vi "AttackerNormal.vi"(4 "AI Parameters":T1={"GotoKick"={"Dist do cone a frente"=150.0, "attacker farback"=1500.0, "Perto"=300.0, "min dist to kick"=150.0, "kick eps"=0.05, "Time to transition"=0.0}, "Attacker"={"CC chute"=0.09, "CC passe"=0.045, "Kick Force"=100.0, "D ball-robot Kick"=200.0, "D ball-robot Pass"=0.3}, "Defender"={"D max"=1700.0, "Vel p/ robô av"=1000.0, "Kick Force"=100.0, "D atk-def"=0.0, "D farback"=0.0}, "Timeout"={"Field/v in x"=6.0, "Dist Robots"=300, "Dist up in y"=300}, "Pose Striker"={"dist"=200.0, "Numeric"=-4.0, "dist 2"=200.0}, "Dist Stop"=300.0, "Distance when ball out"=200, "D central gap "=150.0} {"D central gap" format="%#_13g"; "Dist Stop" format="%#_13g"; "Pose Striker"."Numeric" format="%#_13g"; "Defender"."Kick Force" format="%#_13g"; "Defender"."Vel p/ robô av" format="%#_13g"; "Attacker"."D ball-robot Kick" format="%#_13g"; "Attacker"."Kick Force" format="%#_13g"; "Attacker"."CC passe" format="%#_13g"; "Attacker"."CC chute" format="%#_13g"; "GotoKick"."kick eps" format="%#_13g"; "GotoKick"."min dist to kick" format="%#_13g"; "GotoKick"."Perto" format="%#_13g"; "GotoKick"."attacker farback" format="%#_13g"; "GotoKick"."Dist do cone a frente" format="%#_13g"}, 7 "IA State Input 2":T3, 8 "atacando contra?":bool=TRUE, 9 "balls":T6[](array[typedef])=[{"x"=-974.5169677734375, "y"=-3444.3310546875, "timestamp"=timestamp(2082759045.994995 s since 1904-01-01), "Vel_x"=0.0, "Vel_y"=0.0, "Pos Bola Est"=[]}], 10 "Field Size in":T7={"line_width"=10, "field_length"=9000, "field_width"=6000, "boundary_width"=250, "referee_width"=425, "goal_width"=700, "goal_depth"=180, "goal_wall_width"=20, "center_circle_radius"=500, "defense_radius"=500, "defense_stretch"=350, "free_kick_from_defense_dist"=700, "penalty_spot_from_field_line_dist"=450, "penalty_line_from_spot_dist"=350}, 11 "Robot in":T4={"id"=5, "function"=enum."Attacker", "x"=-983.1382446289062, "y"=-3000.010498046875, "orientation"=-1.5516623258590698, "v_tangent"=0.0, "v_normal"=0.0, "v_ang"=0.0, "kick_x"=0.0, "kick_z"=0.0, "dribble"=FALSE, "Timestamp"=timestamp(2082759045.994995 s since 1904-01-01), "dest_x"=0.0, "dest_y"=0.0, "dest_orientation"=0.0, "estimatives"={"est_v_tangent"=0.0, "est_v_normal"=0.0, "est_vx"=0.0, "est_vy"=0.0, "Pos Robot Est"=[]}, "dest_x_kick"=0.0, "dest_y_kick"=0.0, "Gap Coord"=[], "States"=enum."GoToTangent"}) -> (1 "Next State":T2=enum."GoToTangent", 2 "Robot out":T4={"id"=5, "function"=enum."Attacker", "x"=-983.1382446289062, "y"=-3000.010498046875, "orientation"=-1.5516623258590698, "v_tangent"=0.0001540345015520423, "v_normal"=0.008599927144915481, "v_ang"=0.002668461263266586, "kick_x"=0.0, "kick_z"=0.0, "dribble"=FALSE, "Timestamp"=timestamp(2082759045.994995 s since 1904-01-01), "dest_x"=0.0, "dest_y"=0.0, "dest_orientation"=0.0, "estimatives"={"est_v_tangent"=0.0, "est_v_normal"=0.0, "est_vx"=0.0, "est_vy"=0.0, "Pos Robot Est"=[]}, "dest_x_kick"=0.0, "dest_y_kick"=0.0, "Gap Coord"=[], "States"=enum."GoToTangent"}, 3 "kick \nerror":dbl, 6 "Current States":T2=enum."GoToTangent")   [LabVIEW 2016]
uses:
  Core/AI Robot.ctl
  Functions Enum.ctl
  AttackerStates.ctl
  Core/Field Size.ctl
  Core/AI Ball.ctl
  Core/AI Input.ctl
  Core/AI Judge.ctl
  Command Enum.ctl
  Util/Events/Events.ctl
  AI Parameters.ctl
  <vilib>/Analysis/coordinate.llb/2D Cartesian Coordinate Rotation (Scalar).vi
  <vilib>/Analysis/NI_AALPro.lvlib
panel:
  in  "Cone de chute":dbl=0.9 format="%#_13g"
  out "Boolean":bool
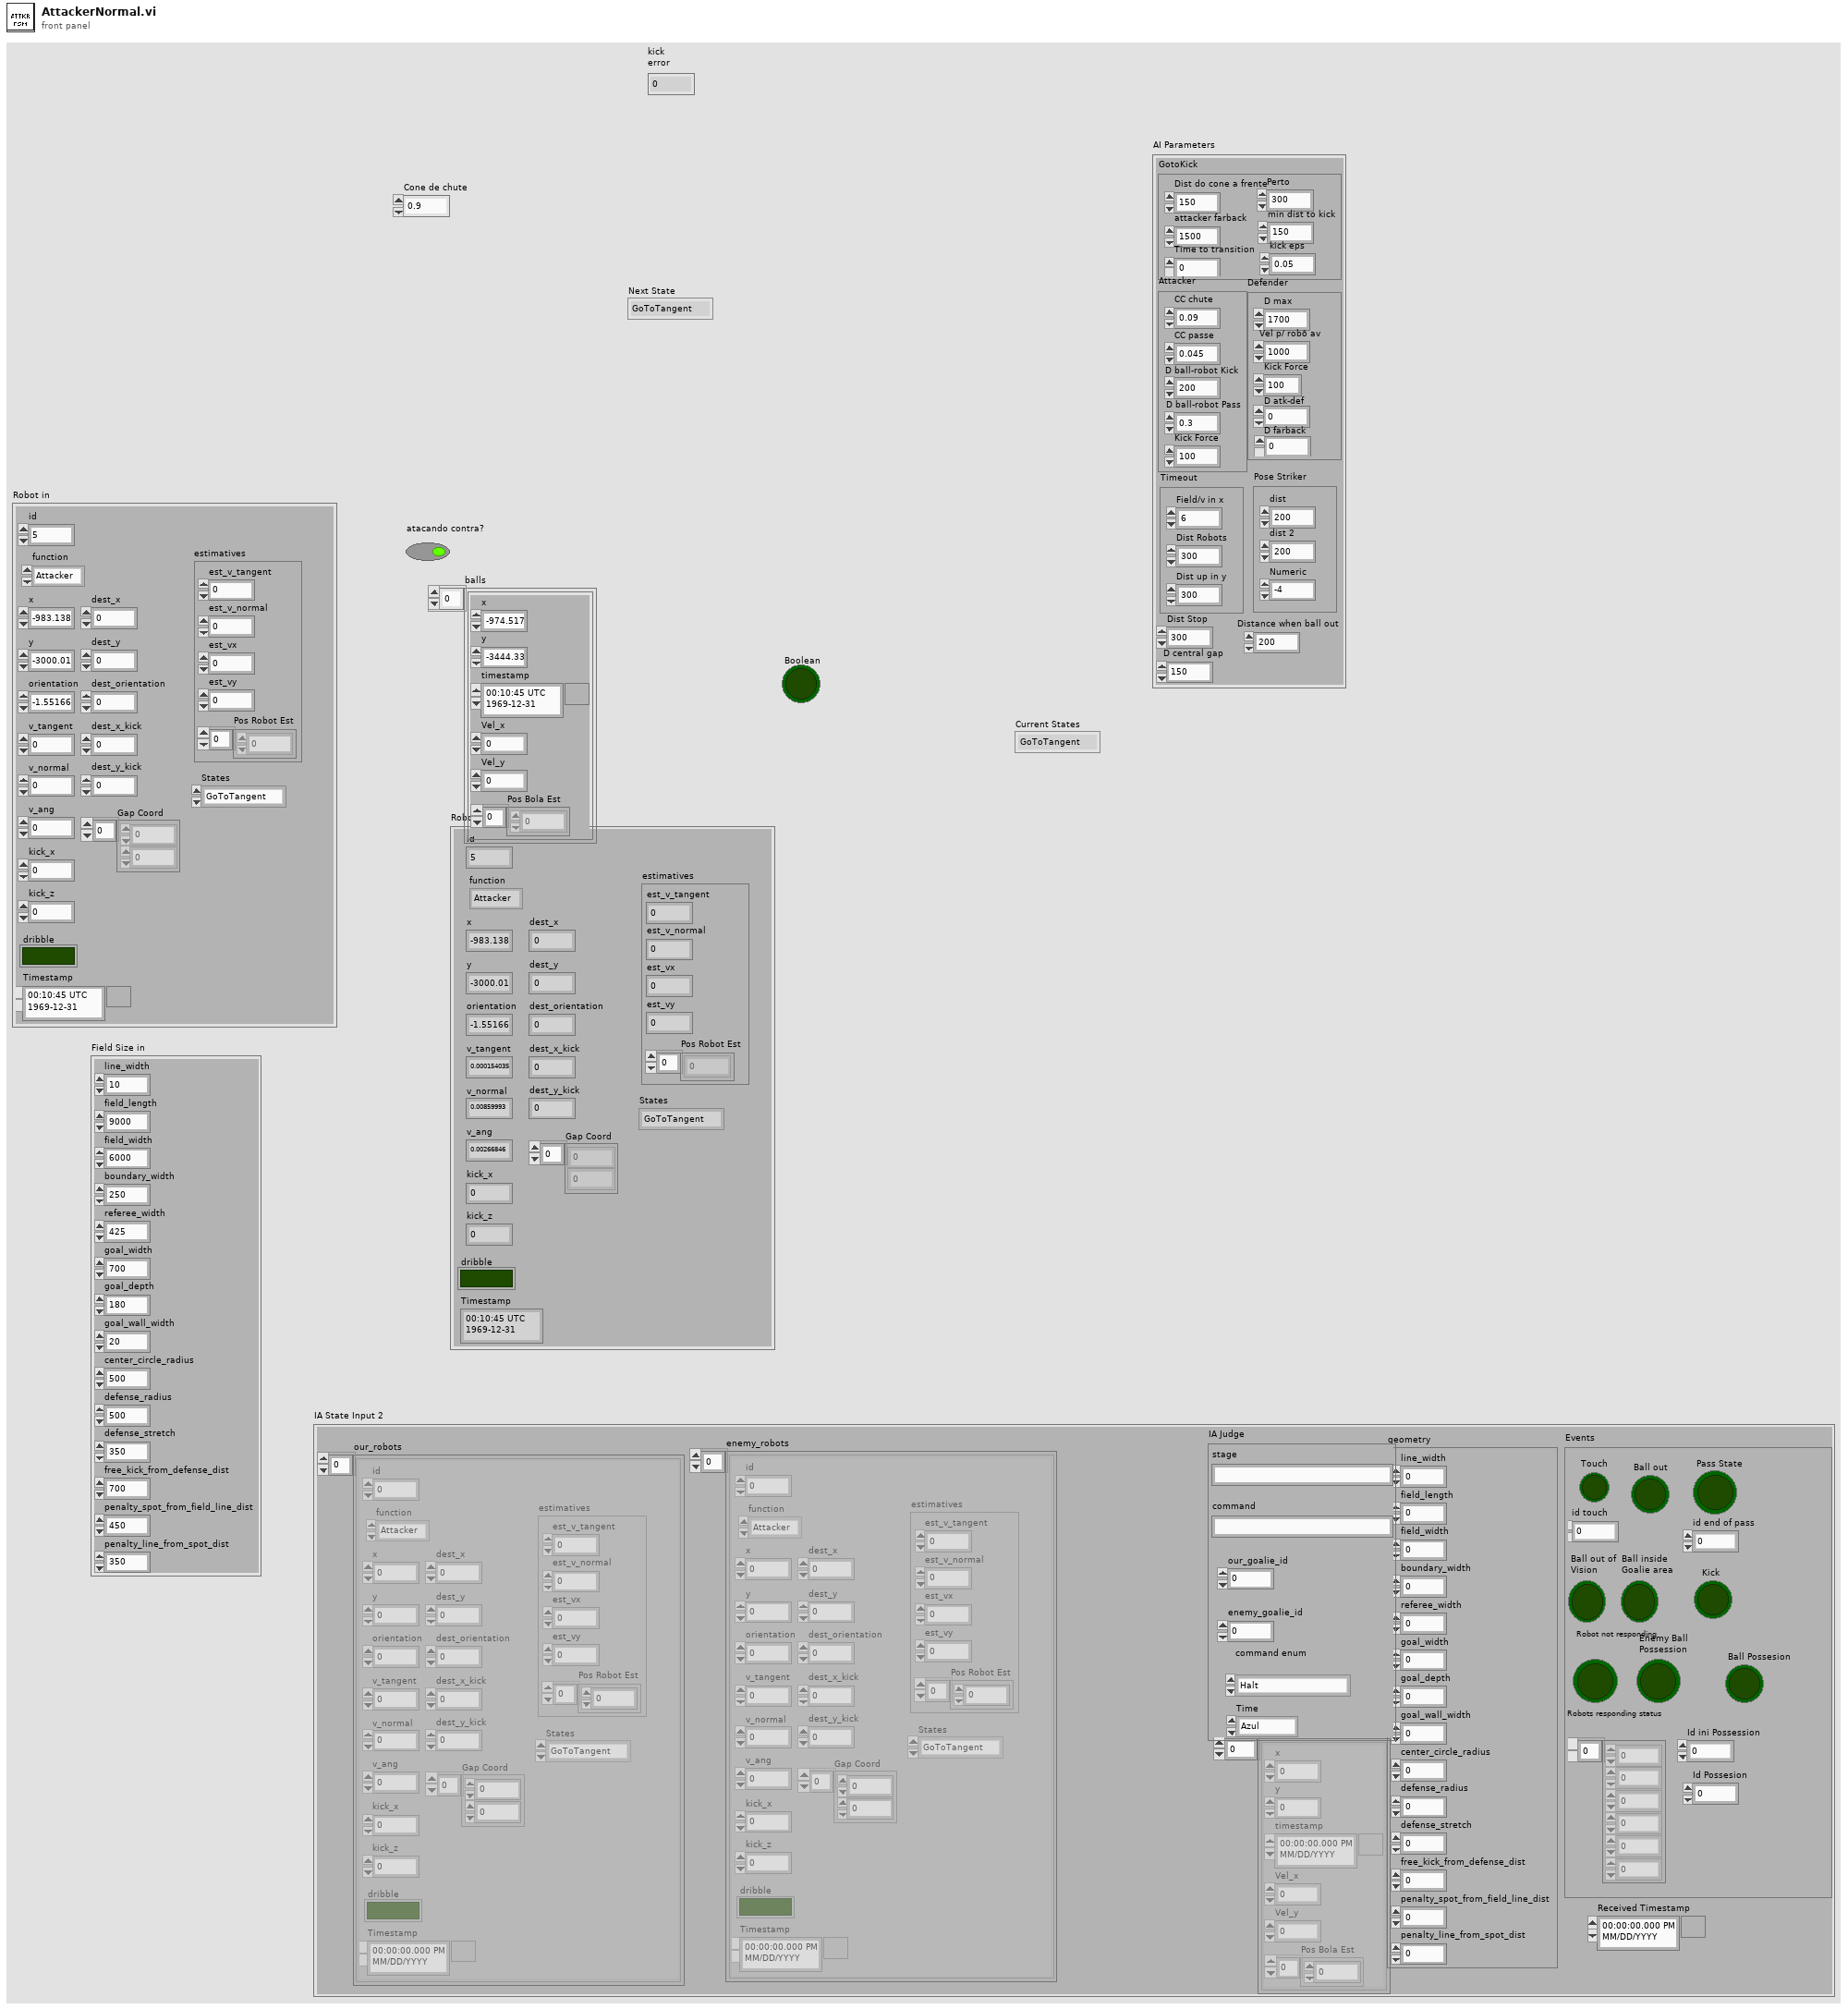
[diagram p1: front panel]
types:
  T1 = typedef "AI Parameters.ctl" = cluster{"GotoKick":cluster{"Dist do cone a frente":dbl, "attacker farback":dbl, "Perto":dbl, "min dist to kick":dbl, "kick eps":dbl, "Time to transition":dbl}, "Attacker":cluster{"CC chute":dbl, "CC passe":dbl, "Kick Force":dbl, "D ball-robot Kick":dbl, "D ball-robot Pass":dbl}, "Defender":cluster{"D max":dbl, "Vel p/ robô av":dbl, "Kick Force":dbl, "D atk-def":dbl, "D farback":dbl}, "Timeout":cluster{"Field/v in x":dbl, "Dist Robots":u32, "Dist up in y":u32}, "Pose Striker":cluster{"dist":dbl, "Numeric":dbl, "dist 2":dbl}, "Dist Stop":dbl, "Distance when ball out":i32, "D central gap ":dbl}
  T2 = typedef "AttackerStates.ctl" = enum16{"Pass", "GoToTangent", "BallGetting", "GoToKick", ""}
  T3 = typedef "AI Input.ctl" = cluster{"our_robots":T4[], "enemy_robots":T4[], "balls":T6[], "geometry":T7, "IA Judge":T8, "Received Timestamp":timestamp, "Events":T10}
  T4 = typedef "AI Robot.ctl" = cluster{"id":u32, "function":T5, "x":dbl, "y":dbl, "orientation":dbl, "v_tangent":dbl, "v_normal":dbl, "v_ang":dbl, "kick_x":dbl, "kick_z":dbl, "dribble":bool, "Timestamp":timestamp, "dest_x":dbl, "dest_y":dbl, "dest_orientation":dbl, "estimatives":cluster{"est_v_tangent":dbl, "est_v_normal":dbl, "est_vx":dbl, "est_vy":dbl, "Pos Robot Est":dbl[]}, "dest_x_kick":dbl, "dest_y_kick":dbl, "Gap Coord":dbl[], "States":T2}
  T5 = typedef "Functions Enum.ctl" = enum16{"Attacker", "Goalie", "Defender", "Striker", "Goto 0", "Dummy", "Kicker", "ZigZag"}
  T6 = typedef "AI Ball.ctl" = cluster{"x":dbl, "y":dbl, "timestamp":timestamp, "Vel_x":dbl, "Vel_y":dbl, "Pos Bola Est":dbl[]}
  T7 = typedef "Field Size.ctl" = cluster{"line_width":u32, "field_length":u32, "field_width":u32, "boundary_width":u32, "referee_width":u32, "goal_width":u32, "goal_depth":u32, "goal_wall_width":u32, "center_circle_radius":u32, "defense_radius":u32, "defense_stretch":u32, "free_kick_from_defense_dist":u32, "penalty_spot_from_field_line_dist":u32, "penalty_line_from_spot_dist":u32}
  T8 = typedef "AI Judge.ctl" = cluster{"stage":string, "command":string, "our_goalie_id":dbl, "enemy_goalie_id":dbl, "command enum":T9, "Time":enum16{"Azul", "Amarelo"}}
  T9 = typedef "Command Enum.ctl" = enum16{"Halt", "Stop", "Force Start", "PKA Normal Start", "Prepare Kickoff Ally", "PKE Normal Start", "Prepare Kickoff Enemy", "Prepare Penalty Ally", "PPA Normal Start", "Prepare Penalty Enemy", "PPE Normal Start", "Direct Free Enemy", "Direct Free Ally", "Indirect Free Enemy", "Indirect Free Ally", "Timeout Enemy", "Timeout Ally", "Goal Enemy", "Goal Ally", "Ball Placement Enemy", "Ball Placement Ally", "Normal Half Time", "Extra Time Break", "Extra Half Time", "None"}
  T10 = typedef "Events.ctl" = cluster{"Touch":bool, "Ball out":bool, "id touch":dbl, "Ball out of \nVision":bool, "Ball inside \nGoalie area":bool, "Robot not responding":bool, "Robots responding status":dbl[], "Enemy Ball \nPossession":bool, "Pass State":bool, "id end of pass":dbl, "Kick":bool, "Id ini Possession":dbl, "Ball Possesion":bool, "Id Possesion":dbl}
  T11 = cluster{"CC chute":dbl, "CC passe":dbl, "Kick Force":dbl, "D ball-robot Kick":dbl, "D ball-robot Pass":dbl}
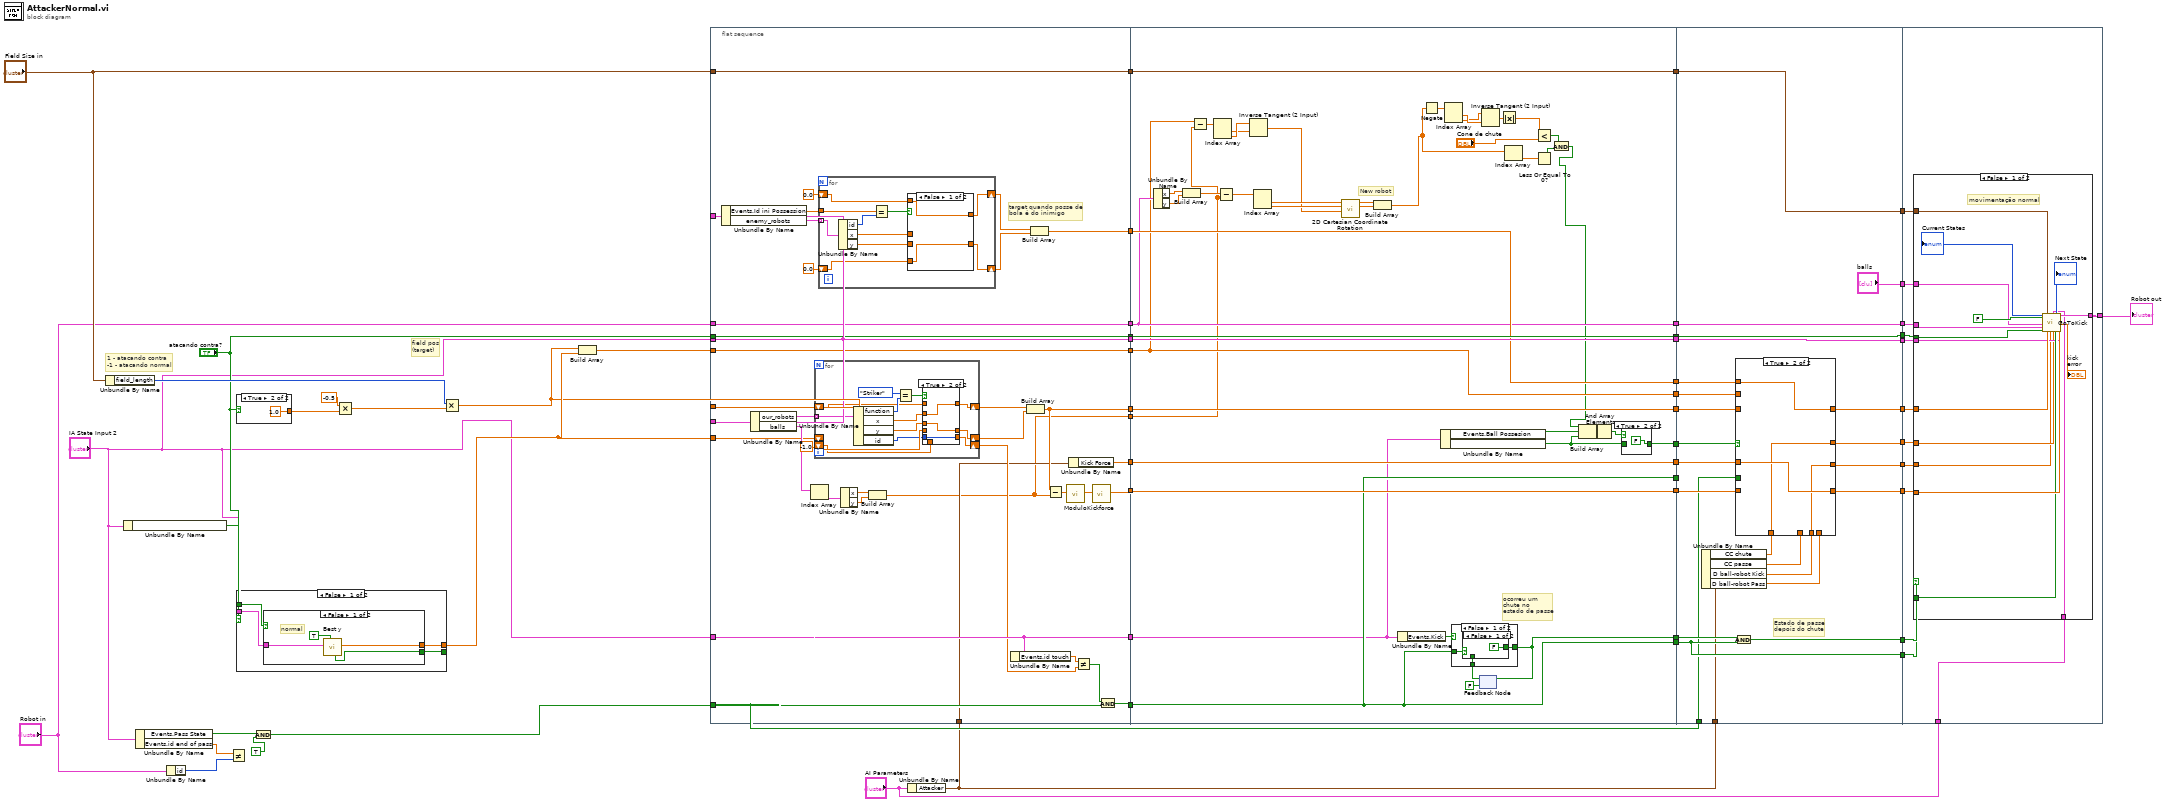
[diagram p0: block diagram]
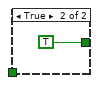
[diagram p6: hidden frame]
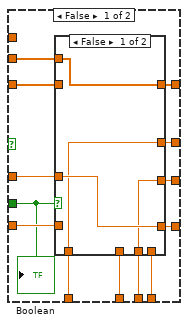
[diagram p7: hidden frame]
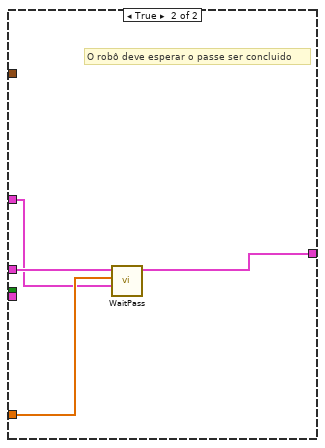
[diagram p9: hidden frame]
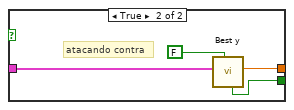
[diagram p10: hidden frame]
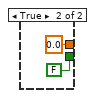
[diagram p11: hidden frame]
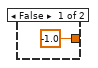
[diagram p12: hidden frame]
diagram:
  # "1 - atacando contra\n-1 - atacando normal"
  # "field pos\n(target)"
  n1 = Unbundle By Name("Field Size in") -> ("field_length"=w56:u32)
  n2 = Unbundle By Name("IA State Input 2") -> ("Events.Ball inside \nGoalie area"=w52:bool)
  n3 = Unbundle By Name("IA State Input 2") -> ("Events.Pass State"=w46:bool, "Events.id end of pass"=w48:dbl)
  n4 = Unbundle By Name("Robot in") -> ("id"=w47:u32)
  n5 = Not Equal?(x=w48, y=w47) -> ()  [unwired: 1 out]
  n6 = case shown="True" "atacando contra?" {
    tunnel: [-1.0 ("attck contra? 2") 1.0] -> w53
    frame False {
    }
    frame True {
    }
  }
  n7 = case shown="False" w52 {
    tunnel: "atacando contra?" -> [w62 _]
    tunnel: [w61 0.0] -> w24
    tunnel: "IA State Input 2" -> [w60 _]
    tunnel: [w59 FALSE ("Eclipse")] -> _
    frame False {
      n8 = case shown="False" w62 {
        tunnel: [w65 w69] -> w61
        tunnel: w60 -> [w63 w68]
        tunnel: [w64 w67] -> w59
        frame False {
          # "normal"
          n9 = call "Best y.vi"("inimigos"=TRUE, "IA State"=w63) -> ("Best y"=w65:dbl, "Eclipse"=w64:bool)  [unwired: 6 in, 2 out]
        }
        frame True {
          # "atacando contra"
          n10 = call "Best y.vi"("inimigos"=FALSE, "IA State"=w68) -> ("Best y"=w69:dbl, "Eclipse"=w67:bool)  [unwired: 6 in, 2 out]
        }
      }
    }
    frame True {
    }
  }
  n11 = And(x=w46, y=TRUE) -> (x .and. y?=w6:bool)
  n12 = Multiply(x=-0.5, y=w53) -> (x*y=w54:dbl)
  n13 = Multiply(x=w56, y=w54) -> (x*y=w23:dbl)
  n14 = Build Array(w23, w24) -> (w45:dbl[])
  n15 = flat-sequence {
    tunnel: "IA State Input 2" -> [w89]
    tunnel: w6 -> [w85]
    tunnel: w23 -> [w91]
    tunnel: w45 -> [w105]
    tunnel: "IA State Input 2" -> [w106]
    tunnel: "Robot in" -> [w107]
    tunnel: "Field Size in" -> [w108]
    tunnel: "atacando contra?" -> [w109]
    tunnel: [w109] -> w33
    tunnel: [w108] -> w32
    tunnel: [w107] -> w31
    tunnel: [w106] -> w30
    tunnel: [w92] -> w29
    tunnel: [w105] -> w28
    tunnel: [w93] -> w27
    tunnel: [w84] -> w26
    tunnel: [w89] -> w25
    tunnel: w24 -> [w95]
    tunnel: "IA State Input 2" -> [w94]
    tunnel: [w74] -> w22
    tunnel: "IA State Input 2" -> [w83]
    tunnel: [w78] -> w17
    tunnel: w4 -> [w75]
    tunnel: [w73] -> w1
    tunnel: [w186] -> w44
    tunnel: [w185] -> w43
    tunnel: [w159] -> w42
    tunnel: [w184] -> w41
    tunnel: [w177] -> w40
    tunnel: [w183] -> w39
    tunnel: [w182] -> w38
    tunnel: [w152] -> w37
    tunnel: [w181] -> w36
    tunnel: [w176] -> w35
    tunnel: [w176] -> w34
    tunnel: w33 -> [w186]
    tunnel: w32 -> [w185]
    tunnel: w31 -> [w159]
    tunnel: w30 -> [w184]
    tunnel: w29 -> [w182]
    tunnel: w28 -> [w152]
    tunnel: w27 -> [w181]
    tunnel: w26 -> [w176]
    tunnel: w25 -> [w175]
    tunnel: w22 -> [w183]
    tunnel: [w144] -> w20
    tunnel: [w174] -> w18
    tunnel: w17 -> [w174]
    tunnel: w1 -> [w151]
    tunnel: w44 -> [w208]
    tunnel: w43 -> [w211]
    tunnel: w42 -> [w210]
    tunnel: w41 -> [w209]
    tunnel: w40 -> [w218]
    tunnel: w39 -> [w217]
    tunnel: w38 -> [w216]
    tunnel: w37 -> [w215]
    tunnel: w36 -> [w214]
    tunnel: w35 -> [w203]
    tunnel: w34 -> [_]
    tunnel: w20 -> [w213]
    tunnel: w18 -> [w212]
    tunnel: [w211] -> w16
    tunnel: [w210] -> w15
    tunnel: [w209] -> w14
    tunnel: [w208] -> w13
    tunnel: [w207] -> w12
    tunnel: [w206] -> w11
    tunnel: [w205] -> w10
    tunnel: [w204] -> w9
    tunnel: [w203] -> w8
    tunnel: w6 -> [w202]
    tunnel: ["balls"] -> w5
    tunnel: w4 -> [w200]
    tunnel: [w196] -> w2
    tunnel: w16 -> [w256]
    tunnel: w15 -> [w255]
    tunnel: w14 -> [w254]
    tunnel: w13 -> [w253]
    tunnel: w12 -> [w252]
    tunnel: w11 -> [w251]
    tunnel: w10 -> [w250]
    tunnel: w9 -> [w249]
    tunnel: w8 -> [w248]
    tunnel: [w247] -> w7
    tunnel: w5 -> [w246]
    tunnel: "AI Parameters" -> [w245]
    tunnel: w2 -> [w244]
    frame #0 {
      # "target quando posse de\nbola é do inimigo"
      n16 = Unbundle By Name(w83) -> ("Events.Id ini Possession"=w81:dbl, "enemy_robots"=w82:T4[])
      n17 = Unbundle By Name(w94) -> ("our_robots"=w96:T4[], "balls"=w99:T6[])
      n18 = Index Array(array=w99) -> (element=w100:T6)  [unwired: 1 in]
      n19 = for {
        tunnel: w96 -> [w136] mode=indexing
        shift-right: [w131] -> w97
        shift-left: w91 -> [w130]
        shift-right: [w128] -> w98
        shift-left: w95 -> [w127]
        shift-right: [w125] -> w87
        shift-left: -1.0 -> [w124]
        n20 = Unbundle By Name(w136) -> ("function"=w135:T5, "x"=w132:dbl, "y"=w129:dbl, "id"=w126:u32)
        n21 = Equal?(x=Functions_Enum."Striker", y=w135) -> (x = y?=w133:bool)
        n22 = case shown="True" w133 {
          tunnel: [w139 w142] -> w131
          tunnel: w132 -> [_ w142]
          tunnel: w130 -> [w139 _]
          tunnel: w129 -> [_ w141]
          tunnel: [w138 w141] -> w128
          tunnel: w127 -> [w138 _]
          tunnel: w126 -> [_ w140]
          tunnel: [w137 w140] -> w125
          tunnel: w124 -> [w137 _]
          frame False {
          }
          frame True {
          }
        }
      }
      n23 = for {
        tunnel: w82 -> [w119] mode=indexing
        tunnel: w81 -> [w117]
        shift-right: [w113] -> w80
        shift-left: 0.0 ("x") -> [w111]
        shift-right: [w112] -> w79
        shift-left: 0.0 ("y") -> [w110]
        n24 = Unbundle By Name(w119) -> ("id"=w118:u32, "x"=w115:dbl, "y"=w114:dbl)
        n25 = Equal?(x=w117, y=w118) -> (x = y?=w116:bool)
        n26 = case shown="False" w116 {
          tunnel: w115 -> [_ w123]
          tunnel: w114 -> [_ w122]
          tunnel: [w121 w123] -> w113
          tunnel: [w120 w122] -> w112
          tunnel: w111 -> [w121 _]
          tunnel: w110 -> [w120 _]
          frame False {
          }
          frame True {
          }
        }
      }
      n27 = Unbundle By Name(w100) -> ("x"=w101:dbl, "y"=w102:dbl)
      n28 = Build Array(w101, w102) -> (w73:dbl[])
      n29 = Unbundle By Name(w89) -> ("Events.id touch"=w88:dbl)
      n30 = Build Array(w97, w98) -> (w93:dbl[])
      n31 = Build Array(w80, w79) -> (w78:dbl[])
      n32 = Subtract(x=w93, y=w73) -> (x-y=w103:dbl[])
      n33 = call "Modulo.vi"("2D vector"=w103) -> ("Modulo"=w104:dbl)  [unwired: 10 in]
      n34 = Unbundle By Name(w75) -> ("Kick Force"=w74:dbl)
      n35 = Not Equal?(x=w88, y=w87) -> (x != y?=w86:bool)
      n36 = call "Kickforce.vi"("Distância ao\nalvo do chute"=w104) -> ("Força do chute"=w92:dbl)  [unwired: 9 in, 1 out]
      n37 = And(x=w86, y=w85) -> (x .and. y?=w84:bool)
    }
    frame #1 {
      # "New robot"
      # "ocorreu um \nchute no\nestado de passe"
      n38 = Unbundle By Name(w159) -> ("x"=w158:dbl, "y"=w157:dbl)
      n39 = Build Array(w158, w157) -> (w156:dbl[])
      n40 = Subtract(x=w152, y=w151) -> (x-y=w153:dbl[])
      n41 = Index Array(array=w153) -> (element #1=w154:dbl, element #2=w155:dbl)  [unwired: 2 in]
      n42 = Subtract(x=w156, y=w151) -> (x-y=w162:dbl[])
      n43 = Inverse Tangent (2 Input)(1:w154, 2:w155) -> (0:w150:dbl)
      n44 = Index Array(array=w162) -> (element #1=w164:dbl, element #2=w163:dbl)  [unwired: 2 in]
      n45 = call-poly <vilib>:"2D Cartesian Coordinate Rotation.vi"("theta"=w150, "y"=w163, "x"=w164) -> ("y out"=w160:dbl, "x out"=w161:dbl)  [unwired: 6 in, 1 out]
      n46 = Build Array(w161, w160) -> (w149:dbl[])
      n47 = Unbundle By Name(w175) -> ("Events.Kick"=w178:bool)
      n48 = Negate(x=w149) -> (-x=w173:dbl[])
      n49 = Unbundle By Name(w175) -> ("Events.Ball Possesion"=w147:bool, "Events.Enemy Ball \nPossession"=w143:bool)
      n50 = Index Array(array=w173) -> (element #1=w172:dbl, element #2=w171:dbl)  [unwired: 2 in]
      n51 = feedback #1(FALSE) -> (w179:bool)
      n52 = case shown="False" w178 {
        tunnel: [w190 TRUE] -> w177
        tunnel: w179 -> [w189 _]
        tunnel: w176 -> [w191 _]
        frame False {
          n53 = case shown="False" w191 {
            tunnel: [FALSE w193] -> w190
            tunnel: w189 -> [_ w193]
            frame False {
            }
            frame True {
            }
          }
        }
        frame True {
        }
      }
      n54 = feedback-in #1(w177) -> ()
      n55 = Inverse Tangent (2 Input)(1:w172, 2:w171) -> (0:w170:dbl)
      n56 = Absolute Value(x=w170) -> (abs(x)=w165:dbl)
      n57 = Index Array(array=w149) -> (element=w168:dbl)  [unwired: 1 in]
      n58 = Less?(x=w165, y="Cone de chute") -> (x < y?=w167:bool)
      n59 = Less Or Equal To 0?(x=w168) -> (x <= 0?=w166:bool)
      n60 = And(x=w167, y=w166) -> (x .and. y?=w146:bool)
      n61 = Build Array(w146, w147, w143) -> (w148:bool[])
      n62 = And Array Elements(Boolean array=w148) -> (logical AND=w145:bool)
      n63 = case shown="True" w145 {
        tunnel: [w187 FALSE] -> w144
        tunnel: w143 -> [w187 _]
        frame False {
        }
        frame True {
        }
      }
    }
    frame #2 {
      # "Estado de passe\ndepois do chute"
      n64 = Unbundle By Name(w200) -> ("CC chute"=w199:dbl, "CC passe"=w198:dbl, "D ball-robot Kick"=w197:dbl, "D ball-robot Pass"=w195:dbl)
      n65 = And(x=w218, y=w203) -> (x .and. y?=w204:bool)
      n66 = case shown="True" w213 {
        tunnel: w217 -> [w231 w243]
        tunnel: w216 -> [w230 _]
        tunnel: w215 -> [w229 _]
        tunnel: w214 -> [w228 _]
        tunnel: [w227 w242] -> w207
        tunnel: [w226 w243] -> w205
        tunnel: w202 -> [w225 _]
        tunnel: w212 -> [_ w242]
        tunnel: [w224 w241] -> w206
        tunnel: w199 -> [w223 w241]
        tunnel: w198 -> [w222 _]
        tunnel: w197 -> [w221 w240]
        tunnel: [w220 w240] -> w196
        tunnel: w195 -> [w219 _]
        frame False {
          n67 = case shown="False" w225 {
            tunnel: w231 -> [w234 _]
            tunnel: w230 -> [_ w238]
            tunnel: w229 -> [w235 _]
            tunnel: w228 -> [_ w239]
            tunnel: [w235 w239] -> w227
            tunnel: [w234 w238] -> w226
            tunnel: [w233 w237] -> w224
            tunnel: w223 -> [w233 _]
            tunnel: w222 -> [_ w237]
            tunnel: [w232 w236] -> w220
            tunnel: w221 -> [w232 _]
            tunnel: w219 -> [_ w236]
            frame False {
            }
            frame True {
            }
          }
          "Boolean" <- w225
        }
        frame True {
        }
      }
    }
    frame #3 {
      n68 = case shown="False" w249 {
        tunnel: w253 -> [w270 _]
        tunnel: w256 -> [w269 _]
        tunnel: w255 -> [w268 w275]
        tunnel: w252 -> [w267 w274]
        tunnel: w250 -> [w266 _]
        tunnel: w248 -> [w265 _]
        tunnel: w254 -> [w264 _]
        tunnel: [w263 w276] -> w247
        tunnel: w251 -> [w261 _]
        tunnel: w246 -> [w260 w273]
        tunnel: w245 -> [w259 _]
        tunnel: w244 -> [w257 _]
        frame False {
          # "movimentação normal"
          n69 = call "GoToKick.vi"("goleiro?"=FALSE, "balls"=w260, "Robot in in"=w268, "atacando contra?"=w270, "Field Size in"=w269, "Target"=w267, "D ball - robot"=w257, "AI Parameters"=w259, "Cone de chute"=w261, "Passe"=w265, "Kick Force"=w266, "IA State Input in"=w264) -> ("Current States"=→"Current States":T2, "Next State"=→"Next State":T2, "Robot out"=w263:T4, "kick error"=→"kick \nerror":dbl)  [unwired: 4 in]
        }
        frame True {
          # "O robô deve esperar o passe ser concluido"
          n70 = call "WaitPass.vi"("balls"=w273, "Target"=w274, "Robot in"=w275) -> ("Robot out"=w276:T4)  [unwired: 8 in]
        }
      }
    }
  }
  n71 = Unbundle By Name("AI Parameters") -> ("Attacker"=w4:T11)
  "Robot out" <- w7
